vi "Test Create Logger with G-CLI Sink.vi"(11 "Test Case In":refnum<class "G-CLI Sink.lvclass">) -> (0 "error out":errorcluster, 3 "Test Case Out":refnum<class "G-CLI Sink.lvclass">)   [LabVIEW 2020, in "G-CLI Sink.lvclass"]
uses:
  G-CLI Sink.lvclass
  C:/Program Files (x86)/National Instruments/LabVIEW 2020/vi.lib/Astemes/LUnit/Test Case.lvclass
  Source/Type Defs/Debug Level.ctl
  <vilib>/Wiresmith Technology/G CLI/CLI Class/CLI.lvclass
  <vilib>/Astemes/LUnit/Test Case.lvclass/Test Case.ctl
  <vilib>/Astemes/LUnit/Core/LUnit Test Case/Private/Append Pass Result.vi
  <vilib>/Astemes/LUnit/Core/LUnit Test Case/Private/Append Fail Result.vi
  <vilib>/Astemes/LUnit/Core/LUnit Test Case/Private/Run In UI.vi
  <vilib>/Utility/error.llb/Clear Errors.vi
  Source/Sinks/G-CLI Sink/G-CLI Sink.lvclass
  C:/Users/hughe_cx/Documents/05_repos/LVLog/Source/Sinks/Sink/Sink.lvclass
  G-CLI Sink.lvclass/G-CLI Sink.ctl
  Source/LV Log.lvlib
  Source/Logger/Logger.lvclass
  <vilib>/Astemes/LUnit/Test Case.lvclass
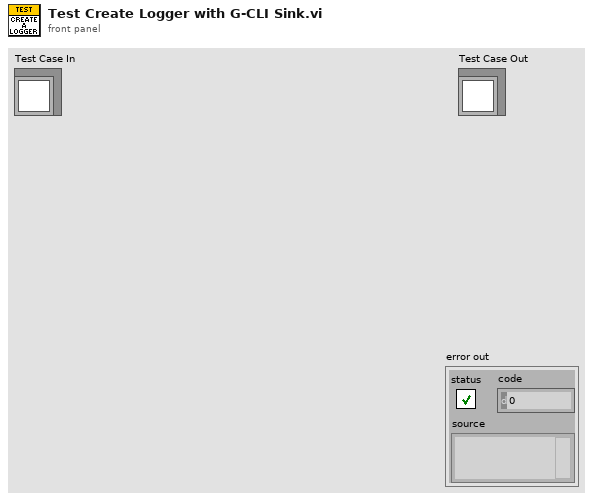
[diagram p1: front panel]
types:
  T1 = typedef "LV Log.lvlib/Debug Level.ctl" = enum16{"DEFAULT", "DEBUG", "INFO", "WARN", "ERROR", "FATAL"}
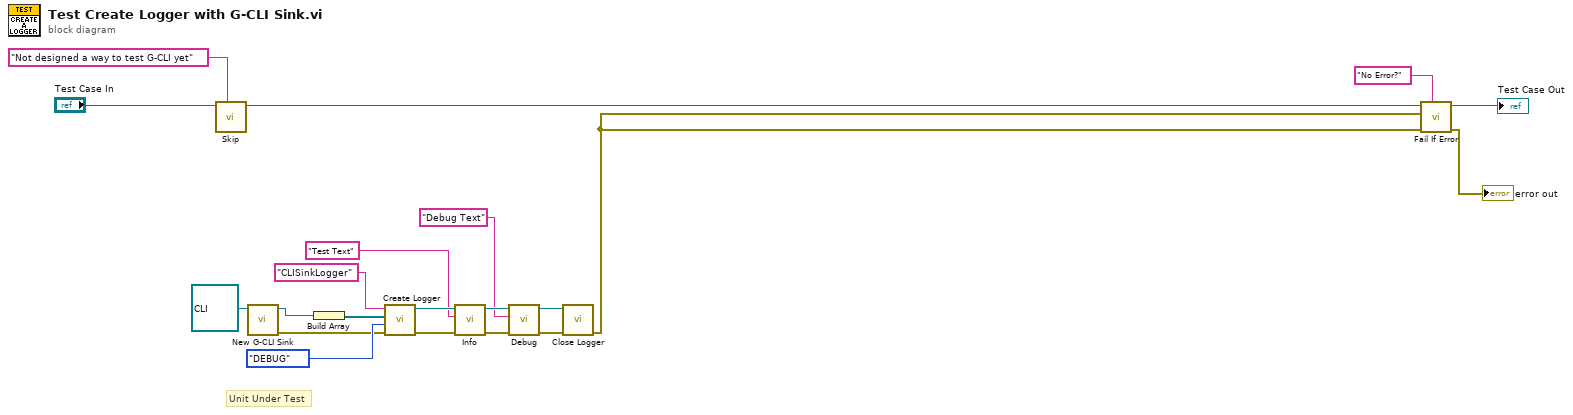
[diagram p0: block diagram]
diagram:
  # "Unit Under Test"
  n1 = call <vilib>:"Skip.vi"("Description"="Not designed a way to test G-CLI yet", "LUnit Test Case In"="Test Case In") -> ("LUnit Test Case Out"=w2:refnum<class "G-CLI Sink.lvclass">)  [unwired: 8 in, 1 out]
  n2 = call "New G-CLI Sink.vi"("CLI Connection"=refnum<class "CLI.lvclass"> refnum) -> ("error out"=w7:errorcluster, "G-CLI Sink out"=w6:refnum<class "G-CLI Sink.lvclass">)  [unwired: 9 in]
  n3 = Build Array(w6) -> (w14:refnum<class "G-CLI Sink.lvclass">[])
  n4 = call "Create Logger.vi"("error in (no error)"=w7, "Debug Level (Default)"=Debug_Level."DEBUG" ("Debug Level in"), "Sinks (Default)"=w14, "Name"="CLISinkLogger") -> ("error out"=w21:errorcluster, "Logger out"=w20:refnum<class "Logger.lvclass">)  [unwired: 6 in]
  n5 = call "Info.vi"("error in (no error)"=w21, "Log Text"="Test Text", "Logger in"=w20) -> ("error out"=w18:errorcluster, "Logger out"=w17:refnum<class "Logger.lvclass">)  [unwired: 6 in, 1 out]
  n6 = call "Debug.vi"("error in (no error)"=w18, "Log Text"="Debug Text", "Logger in"=w17) -> ("error out"=w11:errorcluster, "Logger out"=w10:refnum<class "Logger.lvclass">)  [unwired: 6 in, 1 out]
  n7 = call "Close Logger.vi"("error in (no error)"=w11, "Logger in"=w10) -> ("error out"=w4:errorcluster)  [unwired: 9 in]
  n8 = call <vilib>:"Fail If Error.vi"("Description"="No Error?", "error in (no error)"=w4, "Assert error"=w4, "LUnit Test Case In"=w2) -> ("error out"=→"error out":errorcluster, "LUnit Test Case Out"=→"Test Case Out":refnum<class "G-CLI Sink.lvclass">)  [unwired: 6 in]
